vi "I2C OLEDGestureDemo.vi"() -> ()   [LabVIEW 2020, in "CTI-Scratchpad.lvlib"]
uses:
  CTI-Scratchpad.lvlib
  CTI/Identity.ctl
  CTI/Error Reporting.ctl
  CTI-Peripheral/Gesture Sensor/Base/Gesture.ctl
  CTI/GPIO Number.ctl
  CTI/I2C Number.ctl
  CTI/Session/Session.lvclass
  CTI-Peripheral/Gesture Sensor/Grove Gesture Sensor PAJ7620U2/Grove Gesture Sensor PAJ7620U2.lvclass
  CTI-Peripheral/I2C OLED/64x128 I2C OLED SSD1315/64x128 I2C OLED SSD1315.lvclass
  CTI/VisaComms/VisaComms.lvclass
  CTI/CTI.lvlib
  CTI-Peripheral/Gesture Sensor/Base/Gesture Sensor.lvclass
panel:
  out "Identity":T1
  in  "stop":bool
  out "2D Picture":picture
  in  "Grove Connector":enum16{"I2C0", "I2C1"}(ring)
  out "error out":errorcluster
  in  "Port":refnum<visa-resource-name>="COM4"
  # "https://wiki.seeedstudio.com/Grove-OLED-Display-0.96-SSD1315/"
  # "https://www.seeedstudio.com/Grove-Gesture-PAJ7620U2.html"
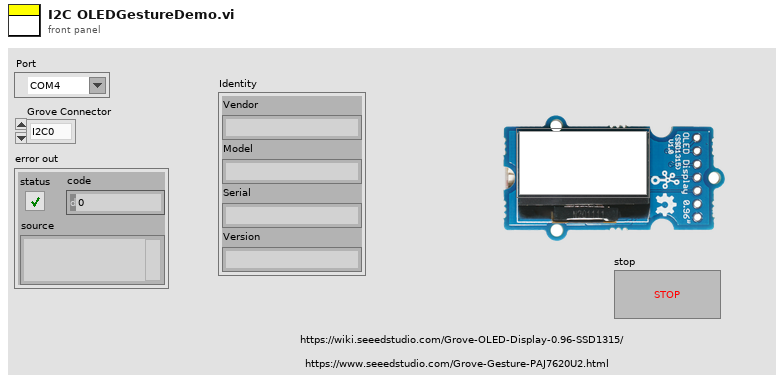
[diagram p1: front panel]
types:
  T1 = typedef "CTI.lvlib/Identity.ctl" = cluster{"Vendor":string, "Model":string, "Serial":string, "Version":string}
  T2 = typedef "CTI-Peripheral.lvlib/Gesture Sensor.lvclass/Gesture.ctl" = enum16{"No Gesture", "Up", "Down", "Left", "Right", "Forward", "Backward", "Clockwise", "Counterclockwise", "Wave"}
  T3 = cluster{"image type":i32, "image depth":i32, "image":u8[], "mask":u8[], "colors":u32[], "Rectangle":cluster{"left":i16, "top":i16, "right":i16, "bottom":i16}}
  T4 = typedef "CTI.lvlib/Error Reporting.ctl" = enum16{"Minimal", "Moderate", "Full"}
  T5 = typedef "CTI.lvlib/I2C Number.ctl" = i8
  T6 = typedef "CTI.lvlib/GPIO Number.ctl" = i8
  T7 = cluster{"image type":i32, "image depth":i32, "image":u8[], "mask":u8[], "colors":u32[], "Rectangle":cluster{"left":i16, "top":i16, "right":i16, "bottom":i16}}[]
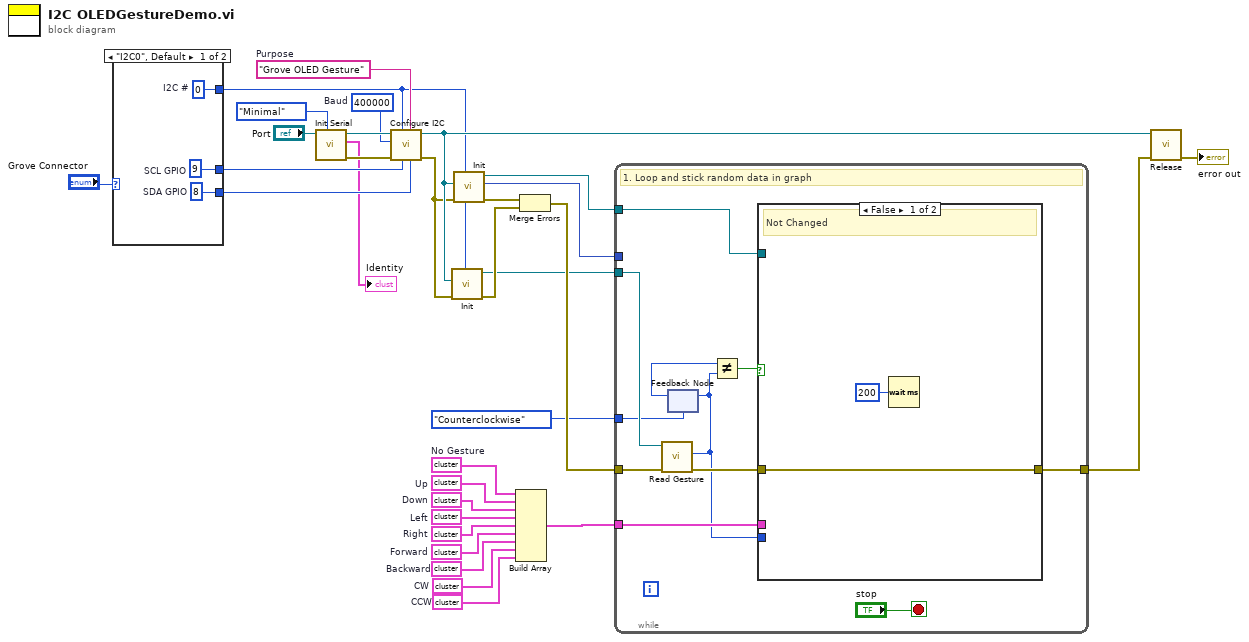
[diagram p0: block diagram]
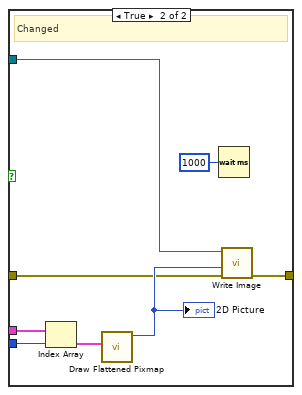
[diagram p2: hidden frame]
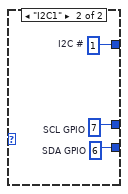
[diagram p3: hidden frame]
diagram:
  w9 = T3 {"image type"=0, "image depth"=8, "image"=array[8192 elements], "mask"=[], "colors"=[16777215, 15461356, 16579836, 11513775, 8158332, 13421772, 13816530, 0, 921102, 15329769, 8553090, 3421236, 15461355, 14935011, 1447446, 10000536, 1052688, 14803425, 15921906, 15000804, 13684944, 15856113, 16645629, 15658734, 3552822, 4079166, 11119017, 8289918, 4276545, 1052687, 395014, 7829367, 12171705, 15527148, 11645361, 65793, 131586, 2763306, 10987431, 16119285, 16316664, 6316128, 197379, 6447714, 14277081, 13158600, 6645093, 11316396, 13224393, 11184810, 6250335, 263172, 2171169, 13948116, 8092539, 10066329, 16250871, 12829635, 6118749, 2434341, 14013909, 16711422, 13750737, 8816262, 9868950, 14869218, 9474192, 4144959, 10658466, 3750201, 4934475, 15987699, 10724259, 328965, 9934743, 15790320, 12237498, 5592405, 15263976, 16185078, 6842472, 789516, 13487565, 7763574, 3815994, 16382457, 16514043, 5921370, 789515, 13092807, 12566463, 3684408, 12632256, 3355443, 11053224, 15592941, 14737632, 14145495, 5197647, 7697781, 14540253, 9408399, 16448250, 12698049, 12369084, 11579568, 14474460, 1644825, 5131854, 15066597, 3158320, 14671839, 4539717, 13355979, 13027014, 11382189, 10197915, 7105644, 15724527, 6974058, 7960953, 9276813, 8026746, 9342606, 4210752, 12303291, 11250603, 13882323, 11776947, 9013641, 8355711, 8882055, 11711154, 15527405, 14343133, 13553358, 14342874, 1907997, 7434609, 394758, 2368548, 5460819, 6710886, 4605510, 6776679, 12895428, 657930, 2302755, 5066061, 4473924, 3158064, 8618883, 2236962, 9079434, 4408131, 14079702, 13290186, 9211020, 7039851, 13619151, 5789784, 4342338, 5987163, 460551, 6513507, 855309, 5000268, 1315860, 12040119, 5526612, 9539985, 4802889, 12105912, 3092271, 986895, 8224125, 9605778, 2829099, 1776411, 7566195, 1381653, 2500134, 15395562, 0, 0, 0, 0, 0, 0, 0, 0, 0, 0, 0, 0, 0, 0, 0, 0, 0, 0, 0, 0, 0, 0, 0, 0, 0, 0, 0, 0, 0, 0, 0, 0, 0, 0, 0, 0, 0, 0, 0, 0, 0, 0, 0, 0, 0, 0, 0, 0, 0, 0, 0, 0, 0, 0, 0, 0, 0, 0, 0, 0, 0, 0, 0, 0, 0, 0, 0, 0, 0, 0, 0, 0, 0], "Rectangle"={"left"=0, "top"=0, "right"=128, "bottom"=64}}  # CCW
  w10 = T3 {"image type"=0, "image depth"=8, "image"=array[8192 elements], "mask"=[], "colors"=[16777215, 15461356, 13421772, 8158332, 11513775, 16579836, 15329769, 921102, 0, 13816530, 15461355, 3421236, 8553090, 10000536, 1447446, 14935011, 16645629, 15856113, 13684944, 15000804, 15921906, 14803425, 1052688, 15527148, 12171705, 7829367, 4079166, 395014, 1052687, 4276545, 8289918, 11119017, 3552822, 15658734, 16119285, 10987431, 2763306, 131586, 65793, 11645361, 14277081, 6447714, 197379, 6316128, 16316664, 13948116, 2171169, 263172, 6250335, 11184810, 13224393, 13158600, 11316396, 6645093, 14013909, 2434341, 6118749, 12829635, 16250871, 10066329, 8092539, 4144959, 9474192, 14869218, 9868950, 8816262, 13750737, 16711422, 9934743, 328965, 10724259, 15987699, 4934475, 3750201, 10658466, 789516, 6842472, 16185078, 15263976, 5592405, 12237498, 15790320, 16382457, 3815994, 7763574, 13487565, 5921370, 16514043, 13092807, 789515, 12566463, 12632256, 3684408, 3355443, 15592941, 11053224, 7697781, 5197647, 14145495, 14737632, 12698049, 16448250, 9408399, 14540253, 5131854, 1644825, 14474460, 11579568, 12369084, 13355979, 4539717, 14671839, 3158320, 15066597, 10197915, 11382189, 13027014, 6974058, 15724527, 7105644, 9342606, 8026746, 9276813, 7960953, 12303291, 4210752, 11250603, 11711154, 8882055, 8355711, 9013641, 11776947, 13882323, 15527405, 14343133, 1907997, 8750469, 14342874, 6776679, 12895428, 7368816, 3092271, 8947848, 3618615, 5066061, 12040119, 4802889, 5789784, 5723991, 526344, 14079702, 13290186, 3487029, 13619151, 9803157, 14408667, 394758, 460551, 4408131, 2894892, 5000268, 986895, 5658198, 12105912, 6513507, 7566195, 1973790, 5526612, 2829099, 1776411, 15395562, 0, 0, 0, 0, 0, 0, 0, 0, 0, 0, 0, 0, 0, 0, 0, 0, 0, 0, 0, 0, 0, 0, 0, 0, 0, 0, 0, 0, 0, 0, 0, 0, 0, 0, 0, 0, 0, 0, 0, 0, 0, 0, 0, 0, 0, 0, 0, 0, 0, 0, 0, 0, 0, 0, 0, 0, 0, 0, 0, 0, 0, 0, 0, 0, 0, 0, 0, 0, 0, 0, 0, 0, 0, 0, 0, 0, 0, 0, 0, 0, 0, 0, 0, 0, 0], "Rectangle"={"left"=0, "top"=0, "right"=128, "bottom"=64}}  # CW
  w11 = T3 {"image type"=0, "image depth"=8, "image"=array[8192 elements], "mask"=[], "colors"=[16777215, 16250871, 15724527, 14935011, 14079702, 13421772, 12961221, 15000804, 15921906, 14145495, 11842740, 9342606, 6381921, 3026478, 0, 2960685, 6447714, 9408399, 15395562, 8092539, 3421236, 3487029, 8026746, 11645361, 5066061, 256, 11579568, 16514043, 6513507, 13487565, 16514299, 15856113, 10658466, 1118481, 263172, 263428, 1052944, 10724259, 8684676, 131586, 15198183, 7434609, 65793, 7368816, 723979, 6513763, 2631976, 10066585, 12237754, 12171961, 12171960, 4539973, 14935267, 4605766, 9013640, 15790320, 9013641, 9211275, 15987699, 15987955, 9277068, 11776947, 9803156, 16119285, 16316664, 262916, 10527135, 16382457, 10790308, 11053480, 11776946, 16645885, 16711422, 11908789, 12040375, 2434597, 10198170, 12895683, 12895684, 13224649, 16711678, 13224393, 12961476, 10395550, 2566184, 4934731, 15066596, 13619407, 13422028, 16382456, 16316920, 13487564, 13684943, 15066597, 9013897, 13882579, 13553613, 13488077, 13816529, 9671571, 16185078, 9868950, 10724258, 16448250, 11316396, 16579835, 197379, 11908532, 11777203, 12369083, 12566463, 12763841, 132098, 7960953, 2698025, 13092806, 13092807, 3026733, 328965, 3224112, 10395806, 10527136, 3421492, 328709, 6513251, 986895, 16579836, 8618883, 7303023, 15329769, 15132390, 657930, 1118737, 3026477, 14211288, 13355979, 14013909, 16645629, 5658198, 1513239, 8224125, 5526612, 2434341, 7039851, 13027014, 4868682, 394758, 11447982, 9276813, 10066329, 16053492, 9539985, 7500402, 10526880, 4079166, 6974058, 11908533, 12303291, 6908265, 2894892, 3684408, 14869218, 2171169, 4737096, 3552822, 3355443, 3881787, 3815994, 15658734, 14606046, 5723991, 3750201, 2565927, 10329501, 10263708, 10855845, 7895160, 8882055, 13816530, 8487297, 13684944, 2829099, 1842204, 4013373, 6579300, 1447446, 8750469, 5131854, 2368548, 3618615, 10461087, 9474192, 14277081, 11184810, 1315860, 6184542, 8947848, 789516, 7763574, 1381653, 12763842, 12105912, 5987163, 1579032, 6776679, 15527148, 1907997, 0, 0, 0, 0, 0, 0, 0, 0, 0, 0, 0, 0, 0, 0, 0, 0, 0, 0, 0, 0, 0, 0, 0, 0, 0, 0, 0, 0, 0, 0, 0, 0, 0, 0, 0, 0, 0, 0, 0, 0, 0, 0, 0, 0, 0, 0, 0, 0, 0], "Rectangle"={"left"=0, "top"=0, "right"=128, "bottom"=64}}  # Backward
  w12 = T3 {"image type"=0, "image depth"=8, "image"=array[8192 elements], "mask"=[], "colors"=[16777215, 16250871, 15724527, 15000804, 14079702, 13421772, 12961221, 13355979, 14013909, 14935011, 15921906, 14145495, 11842740, 9408399, 6447714, 3026477, 0, 3026478, 9342606, 14211288, 15395562, 8026746, 3487029, 3421236, 11645361, 5066061, 16514043, 13487565, 6513507, 15856113, 10724259, 657930, 263172, 1118737, 10658466, 8684676, 131586, 8618883, 15329769, 15198183, 7368816, 65793, 7303023, 15132390, 16579836, 256, 1118481, 986895, 6513251, 11579568, 197379, 328965, 3224112, 10395806, 10527136, 3421492, 328709, 2698025, 13092806, 13092807, 3026733, 12566463, 12763841, 132098, 7960953, 12369083, 16711422, 11908532, 11777203, 11776947, 11316396, 16579835, 10724258, 16448250, 6381921, 2960685, 10066585, 9868950, 9671571, 16185078, 9013897, 13882579, 13553613, 13488077, 13816529, 9013641, 4934731, 15066596, 13619407, 13422028, 16382456, 16316920, 13487564, 13684943, 15066597, 2434597, 10198170, 12895683, 12895684, 11908789, 13224649, 16711678, 13224393, 12961476, 10395550, 2566184, 12040375, 11776946, 16645885, 11053480, 16514299, 10527135, 16382457, 10790308, 9803156, 16119285, 16316664, 262916, 9211275, 15987699, 15987955, 9277068, 9013640, 15790320, 4539973, 14935267, 4605766, 2631976, 12237754, 12171961, 12171960, 6513763, 723979, 7434609, 263428, 1052944, 8092539, 16645629, 15263976, 1776411, 5658198, 6052956, 3355443, 2434341, 15527148, 5395026, 10197915, 7105644, 9474192, 15461355, 8750469, 8553090, 8289918, 8882055, 11908533, 7895160, 3618615, 12698049, 7039851, 4013373, 11053224, 723723, 5329233, 1315860, 1513239, 14671839, 12829635, 3289650, 5460819, 14606046, 11513775, 2763306, 7566195, 6776679, 5921370, 3552822, 5855577, 5789784, 921102, 7171437, 7237230, 11184810, 2368548, 7763574, 13027014, 4276545, 15658734, 1579032, 14803425, 1907997, 2565927, 6579300, 10855845, 11711154, 6908265, 3750201, 8224125, 8816262, 2500134, 10921638, 460551, 6316128, 6118749, 5723991, 14277081, 12632256, 7829367, 2631720, 1644825, 10329501, 4934475, 14474460, 3947580, 4539717, 10132122, 1710618, 5592405, 14737632, 5131854, 10790052, 526344, 4605510, 3815994, 12303291, 2894892, 3881787, 4079166, 5197647, 6184542, 10987431, 12040119, 9737364, 855309, 10000536, 4737096, 13750737, 789516, 5000268, 8355711, 0, 0, 0, 0, 0, 0, 0, 0, 0, 0, 0, 0, 0, 0, 0, 0, 0], "Rectangle"={"left"=0, "top"=0, "right"=128, "bottom"=64}}  # Forward
  w13 = T3 {"image type"=0, "image depth"=24, "image"=array[24576 elements], "mask"=[], "colors"=[], "Rectangle"={"left"=0, "top"=0, "right"=128, "bottom"=64}}  # Right
  w14 = T3 {"image type"=0, "image depth"=24, "image"=array[24576 elements], "mask"=[], "colors"=[], "Rectangle"={"left"=0, "top"=0, "right"=128, "bottom"=64}}  # Left
  w15 = T3 {"image type"=0, "image depth"=24, "image"=array[24576 elements], "mask"=[], "colors"=[], "Rectangle"={"left"=0, "top"=0, "right"=128, "bottom"=64}}  # Down
  w16 = T3 {"image type"=0, "image depth"=24, "image"=array[24576 elements], "mask"=[], "colors"=[], "Rectangle"={"left"=0, "top"=0, "right"=128, "bottom"=64}}  # Up
  w17 = T3 {"image type"=0, "image depth"=8, "image"=array[8192 elements], "mask"=[], "colors"=[16777215, 16645629, 14869218, 7237230, 16579836, 14342874, 15592941, 11316396, 3750201, 10395294, 1776411, 5921370, 11250603, 16514043, 7500402, 6513507, 11447982, 13619151, 11776947, 0, 13158600, 5592405, 13224393, 15790320, 12171705, 16711422, 5658198, 14474460, 15658734, 5789784, 2368548, 13948116, 14277081, 13882323, 8750469, 8421504, 16316664, 12237498, 12369084, 14935011, 12105912, 11711154, 12763842, 15066597, 12303291, 11579568, 13421772, 9737364, 9803157, 15198183, 4671303, 13750737, 12434877, 16382457, 5329233, 4737096, 5460819, 5723991, 15856113, 16448250, 11053224, 14540253, 12698049, 13027014, 6250335, 13487565, 131586, 7105644, 65793, 1907997, 13355979, 15921906, 8816262, 11184810, 460551, 4473924, 5131854, 4013373, 14079702, 723723, 8553090, 11513775, 11842740, 5395026, 13816530, 10790052, 8487297, 4539717, 1315860, 2302755, 6184542, 16119285, 9539985, 2434341, 5263440, 13290186, 15000804, 9211020, 6447714, 7434609, 12566463, 6842472, 9934743, 11645361, 6579300, 6381921, 3618615, 10658466, 15461355, 6710886, 6974058, 7895160, 11119017, 11974326, 10855845, 13092807, 263172, 8947848, 9145227, 4802889, 1842204, 15527148, 6645093, 15132390, 4868682, 10724259, 9474192, 15987699, 7631988, 2500134, 16250871, 197379, 5987163, 4079166, 3552822, 13553358, 4408131, 1513239, 328965, 5066061, 7697781, 4934475, 394758, 789516, 1052688, 1381653, 9868950, 12500670, 2171169, 2236962, 1579032, 1973790, 15263976, 10197915, 1447446, 2565927, 3026478, 8882055, 7303023, 14013909, 6908265, 14211288, 5000268, 12632256, 14803425, 14606046, 15395562, 7171437, 1250067, 15724527, 4605510, 4342338, 7566195, 9013641, 10263708, 15329769, 8092539, 14737632, 8684676, 13684944, 7368816, 11908533, 11382189, 4276545, 5197647, 6052956, 9079434, 4210752, 2631720, 526344, 8026746, 3684408, 3487029, 9408399, 3947580, 12961221, 4144959, 2894892, 7039851, 8618883, 3289650, 8289918, 10987431, 5526612, 3815994, 3223857, 2697513, 9342606, 16053492, 3881787, 1644825, 10132122, 3355443, 10066329, 2105376, 1710618, 10461087, 5855577, 1184274, 12829635, 921102, 2039583, 2829099, 657930, 1118481, 2763306, 8158332, 855309, 10921638, 14671839, 0, 0, 0, 0, 0, 0, 0, 0, 0, 0, 0, 0, 0, 0, 0, 0, 0, 0, 0, 0, 0, 0, 0, 0, 0, 0], "Rectangle"={"left"=0, "top"=0, "right"=128, "bottom"=64}}  # No Gesture
  w27 = "Grove OLED Gesture"  # Purpose
  w28 = u32 400000  # Baud
  n1 = case shown="\"I2C0\", Default" "Grove Connector" {
    tunnel: [w35 w38] -> w25
    tunnel: [w34 w37] -> w24
    tunnel: [w33 w36] -> w6
    frame "I2C0", Default {
      w33 = T5 0  # I2C #
      w34 = T6 8  # SDA GPIO
      w35 = T6 9  # SCL GPIO
    }
    frame "I2C1" {
      w36 = T5 1  # I2C #
      w37 = T6 6  # SDA GPIO
      w38 = T6 7  # SCL GPIO
    }
  }
  n2 = call "Init Serial.vi"("Error Checking (Full)"=Error_Reporting."Minimal", "VISA resource name in"="Port") -> ("error out"=w29:errorcluster, "Identity"=→"Identity":T1, "Session"=w30:refnum<class "Session.lvclass">)  [unwired: 7 in]
  n3 = call "Configure I2C.vi"("SDA GPIO"=w24, "Purpose (\"I2C\")"=w27, "SCL GPIO"=w25, "I2C #"=w6, "error in (no error)"=w29, "Baud"=w28, "Session in"=w30) -> ("error out"=w5:errorcluster, "Session out"=w7:refnum<class "Session.lvclass">)  [unwired: 3 in]
  n4 = call "Init.vi"("I2C #"=w6, "error in (no error)"=w5, "Session In"=w7) -> ("error out"=w3:errorcluster, "Grove Gesture Sensor PAJ7620U2 Out"=w2:refnum<class "Grove Gesture Sensor PAJ7620U2.lvclass">)  [unwired: 7 in]
  n5 = call "Init.vi"("I2C #"=w6, "error in (no error)"=w5, "Session In"=w7) -> ("error out"=w20:errorcluster, "2D Picture"=w22:picture, "64x128 I2C OLED SSD1315 Out"=w21:refnum<class "64x128 I2C OLED SSD1315.lvclass">)  [unwired: 6 in]
  n6 = Build Array(w17, w16, w15, w14, w13, w12, w11, w10, w9) -> (w8:T7)
  n7 = Merge Errors(w20, w3) -> (w4:errorcluster)
  n8 = while {
    tunnel: w22 -> [_]
    tunnel: w4 -> [w45]
    tunnel: w21 -> [w49]
    tunnel: [w48] -> w19
    tunnel: w8 -> [w46]
    tunnel: w2 -> [w44]
    tunnel: Gesture."Counterclockwise" ("Gesture") -> [w39]
    stop <- "stop" stop-if-true
    # "1. Loop and stick random data in graph"
    n9 = call-dynamic "Read Gesture.vi"("error in (no error)"=w45, "Grove Gesture Sensor PAJ7620U2 in"=w44) -> ("error out"=w43:errorcluster, "Gesture"=w42:T2)  [unwired: 7 in, 1 out]
    n10 = feedback-in #1(w42) -> ()
    n11 = feedback #1(w39) -> (w41:T2)
    n12 = Not Equal?(x=w41, y=w42) -> (x != y?=w40:bool)
    n13 = case shown="False" w40 {
      tunnel: w49 -> [_ w59]
      tunnel: [w51 w58] -> w48
      tunnel: w46 -> [_ w56]
      tunnel: w43 -> [w51 w54]
      tunnel: w42 -> [_ w53]
      frame False {
        # "Not Changed"
        n14 = Wait (ms)(milliseconds to wait=u32 200) -> ()  [unwired: 1 out]
      }
      frame True {
        # "Changed"
        n15 = Index Array(array=w56, index=w53) -> (element=w57:T3)
        n16 = call <vilib>:"Draw Flattened Pixmap.vi"("image data"=w57) -> ("new picture"=w55:picture)  [unwired: 8 in]
        "2D Picture" <- w55
        n17 = Wait (ms)(milliseconds to wait=u32 1000) -> ()  [unwired: 1 out]
        n18 = call-dynamic "Write Image.vi"("error in (no error)"=w54, "2D Picture"=w55, "64x128 I2C OLED SSD1315 In"=w59) -> ("error out"=w58:errorcluster)  [unwired: 7 in, 1 out]
      }
    }
  }
  n19 = call-dynamic "Release.vi"("error in (no error)"=w19, "Session in"=w7) -> ("error out"=→"error out":errorcluster)  [unwired: 9 in]
